vi "Extract Valid Waypoints.vi"(8 "Bearing":dbl, 9 "Origin Point":T1 {"Latitude" format="%#_10g"; "Longitude" format="%#_10g"}, 10 "Y intersects":dbl[](array[numeric]), 11 "X Intersects":dbl[](array[numeric])) -> (3 "Valid Points":T1[](array[typedef]) {"Latitude" format="%#_10g"; "Longitude" format="%#_10g"})   [LabVIEW 2014]
uses:
  Lat Long Conversion/Controls/PointLatLon.ctl
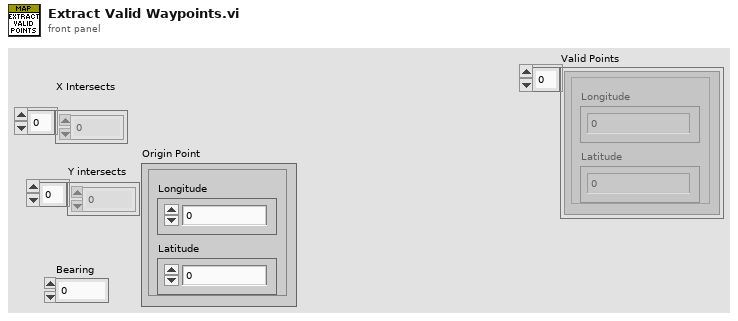
[diagram p1: front panel]
types:
  T1 = typedef "PointLatLon.ctl" = cluster{"Longitude":dbl, "Latitude":dbl}
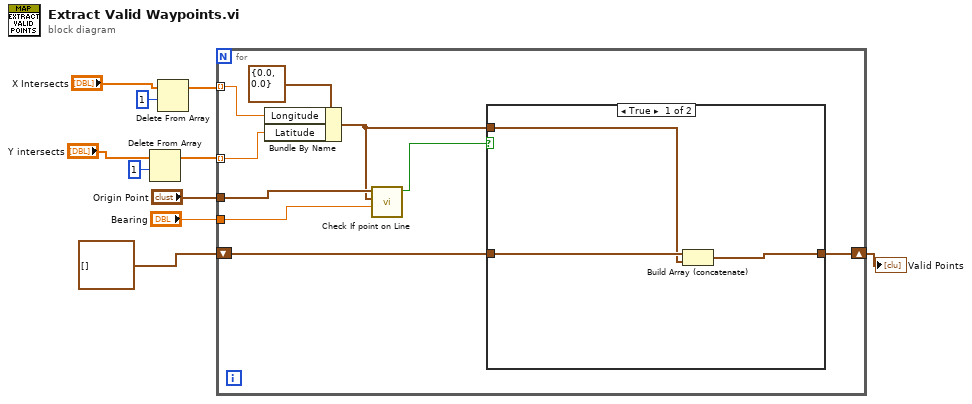
[diagram p0: block diagram]
diagram:
  n1 = Delete From Array(array="Y intersects", length=1) -> (array with subset deleted=w4:dbl[])  [unwired: 1 in, 1 out]
  n2 = Delete From Array(array="X Intersects", length=1) -> (array with subset deleted=w6:dbl[])  [unwired: 1 in, 1 out]
  n3 = for {
    tunnel: w6 -> [w17] mode=indexing
    tunnel: w4 -> [w16] mode=indexing
    shift-right: [w13] -> w9
    shift-left: T1[] [] -> [w19]
    tunnel: "Origin Point" -> [w15]
    tunnel: "Bearing" -> [w14]
    n4 = Bundle By Name(cluster=T1 {"Longitude"=0.0, "Latitude"=0.0} ("Origin Point"), "Longitude"=w17, "Latitude"=w16) -> (w12:T1)
    n5 = call "Check If point on Line.vi"("Original Bearing"=w14, "Point in question"=w12, "Origin Point"=w15) -> ("In Range?"=w11:bool)  [unwired: 7 in, 1 out]
    n6 = case shown="True" w11 {
      tunnel: w19 -> [w22 w23]
      tunnel: [w21 w23] -> w13
      tunnel: w12 -> [w20 _]
      frame True {
        n7 = Build Array (concatenate)(w22, w20) -> (w21:T1[])
      }
      frame False {
      }
    }
  }
  "Valid Points" <- w9
